vi "9082 NIVS FPGA personality + 9862_9862_SEA9811_9220_IO_sim.vi"() -> ()   [LabVIEW 2012]
uses:
  <vilib>/Platform/TimedLoop/XDataNode/timing_clust.ctl
  <vilib>/Platform/TimedLoop/XDataNode/nitl_modes.ctl
  <vilib>/Platform/TimedLoop/XDataNode/wakeup.ctl
  <vilib>/rvi/Emulation/niFpgaSctlEmulationGetInTimedLoop.vi
  <vilib>/rvi/Emulation/niFpgaSctlEmulationGlobalWrite.vi
  <vilib>/rvi/interface/RandomDataEmulation/nirviRandomDataFPGAFIFO.vi
  <vilib>/rvi/interface/RandomDataEmulation/niFpgaRandomDataHandleErrors.vi
  <vilib>/rvi/Emulation/niFpgaSctlEmulationRegisterWithScheduler.vi
  <vilib>/rvi/Emulation/niFpgaSctlEmulationScheduler.vi
  <vilib>/rvi/eio/common/nirviEmuTemplateMethod_errors.vi
  <vilib>/Platform/TimedLoop/XDataNode/XDataNode.xnode
  <vilib>/rvi/DataTransferAndStorage/Container/XNode/niFpgaContainer.xnode
  <vilib>/rvi/interface/RandomDataEmulation/nirviRandomDataFpgaReadWriteTemplate.vi
  <vilib>/eio/EIONode/EIONode.xnode
  <vilib>/Platform/TimedLoop/XDataNode/XDNodeRunTimeDep.lvlib
  <vilib>/NI Veristand/FPGA/NI_VS FPGA Support.lvlib
  <userlib>/_NI VeriStand FPGA Support/NI VeriStand FPGA Clock Support/NI_VS FPGA Clock Support.lvlib
  <vilib>/eio/EIOMethodNode/EIOMethodNode.xnode
  <userlib>/FPGA Timekeeper 1.1b0/FPGA Timekeeper.lvlib
  <vilib>/eio/EIOPropertyNode/EIOPropertyNode.xnode
  <vilib>/rvi/eio/common/nirviEmuTemplatePropertyGet_errors.vi
  <vilib>/rvi/eio/common/nirviEmuTemplatePropertyGet_noerrors.vi
  <vilib>/rvi/eio/common/nirviEmuTemplatePropertySet_errors.vi
  <vilib>/rvi/eio/common/nirviEmuTemplatePropertySet_noerrors.vi
panel:
  out "element":u64
  out "9220/AI0":fxp<+/-,24,5>
  out "Counter":u32
  out "Pulse":bool
  in  "Pulse length (ms)":u32=5
  in  "AI0_threshold (V)":fxp<+/-,24,5>=5.0
  in  "FPGA Loop rate (usec)":u16=5
  out "FPGA Timekeeper time (ns)":u64
  out "FPGA Timekeeper locked":bool
  out "offset from RT time (ns)":i32
  in  "RT time (ns)":u64
  out "DMA Overflow":bool
  out "Elements in FIFO":u32
  out "Rx Status":u16 format="%016b"
  out "Rx rate us":u32
  in  "RxSimRate(mSec)":u32=5 caption="Count(mSec)"
  out "Tx Status":u8 format="%08b"
  in  "Tx Data":u32 format="%08x"
  in  "Transmit Data":bool
  in  "Rx Channel Number":u8 max=7 step=1
  in  "Rx Config Data (RCR)":u16=32 format="%04x"
  in  "Tx Config Data (TCR)":u16=8192 format="%04x"
  in  "Rx Label Filter":u8[](array[numeric])=[0, 0, 0, 0, 0, 0, 0, 0, 0, 0, 0, 0, 0, 0, 0, 0]
  in  "Configure\nchannel":bool
  in  "Finished config":bool
  in  "Generate IRQ":bool
  in  "Use External Timing":bool
  in  "Write to  RTSI":bool
  in  "Loop Rate (usec)":u32
  in  "Start":bool
  # "Configuration"
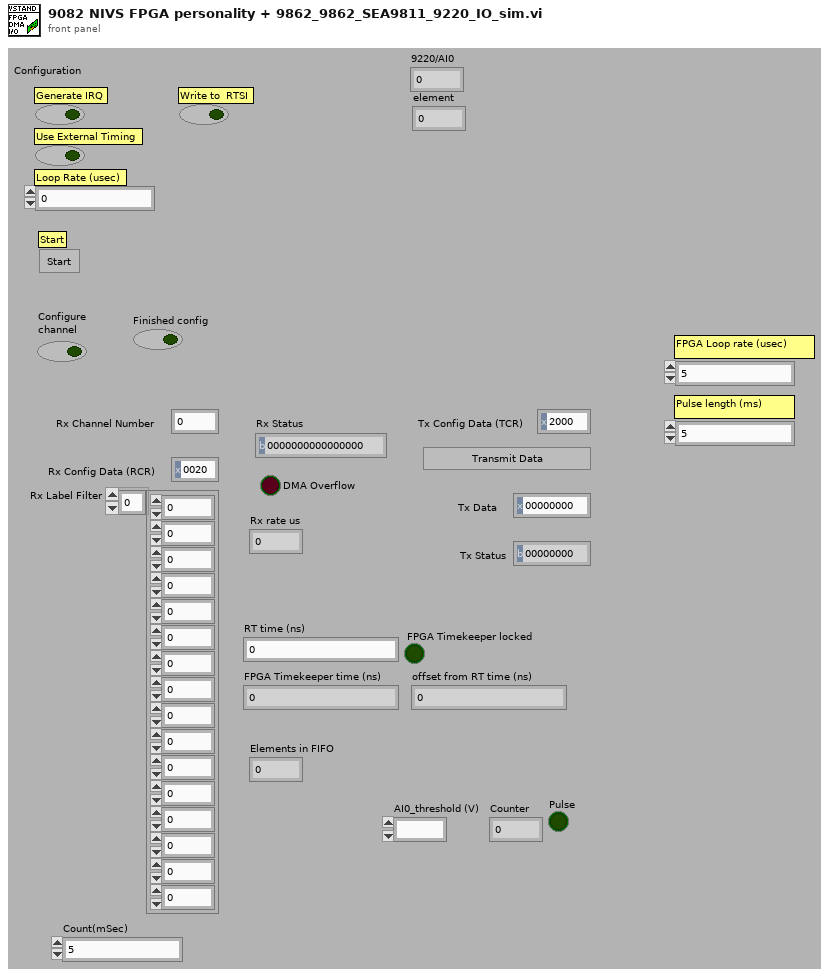
[diagram p1: front panel]
types:
  T1 = typedef "XDNodeRunTimeDep.lvlib/timing_clust.ctl" = cluster{"Expected End [f-1]":u64, "Actual End [f-1]":u64, "Finished Late? [f-1]":bool, "Expected End [i-1]":u64, "Actual End [i-1]":u64, "Finished Late? [i-1]":bool, "Expected Start [i]":u64, "Actual Start [i]":u64, "Expected Start [f]":u64, "Actual Start [f]":u64, "Source Name":string, "Structure Name":string, "Period":i64, "Deadline":i64, "Offset":i64, "Start":i64, "Priority":i32, "Timeout":i32, "Mode":T2, "Wakeup Reason":T3, "Error":errorcluster, "Source Type":string, "Secondary Source Type":string, "Global End Time":u64, "Global Start Time":u64, "Frame Duration":u64, "Iteration Duration":u64, "Assigned CPU":i32, "I/O Scan Engine Mode":u32}
  T2 = typedef "XDNodeRunTimeDep.lvlib/nitl_modes.ctl" = enum32{"No Change", "Process missed periods, maintain original phase", "Discard missed periods, maintain original phase", "Process missed periods, ignore original phase", "Discard missed periods, ignore original phase"}
  T3 = typedef "XDNodeRunTimeDep.lvlib/wakeup.ctl" = enum32{"Normal", "Aborted", "Asynchronous wakeup", "Timing source error", "Timed loop error", "Timeout"}
  T4 = cluster{"Rx Label Filter[0]":u8, "Rx Label Filter[1]":u8, "Rx Label Filter[2]":u8, "Rx Label Filter[3]":u8, "Rx Label Filter[4]":u8, "Rx Label Filter[5]":u8, "Rx Label Filter[6]":u8, "Rx Label Filter[7]":u8, "Rx Label Filter[8]":u8, "Rx Label Filter[9]":u8, "Rx Label Filter[10]":u8, "Rx Label Filter[11]":u8, "Rx Label Filter[12]":u8, "Rx Label Filter[13]":u8, "Rx Label Filter[14]":u8, "Rx Label Filter[15]":u8}
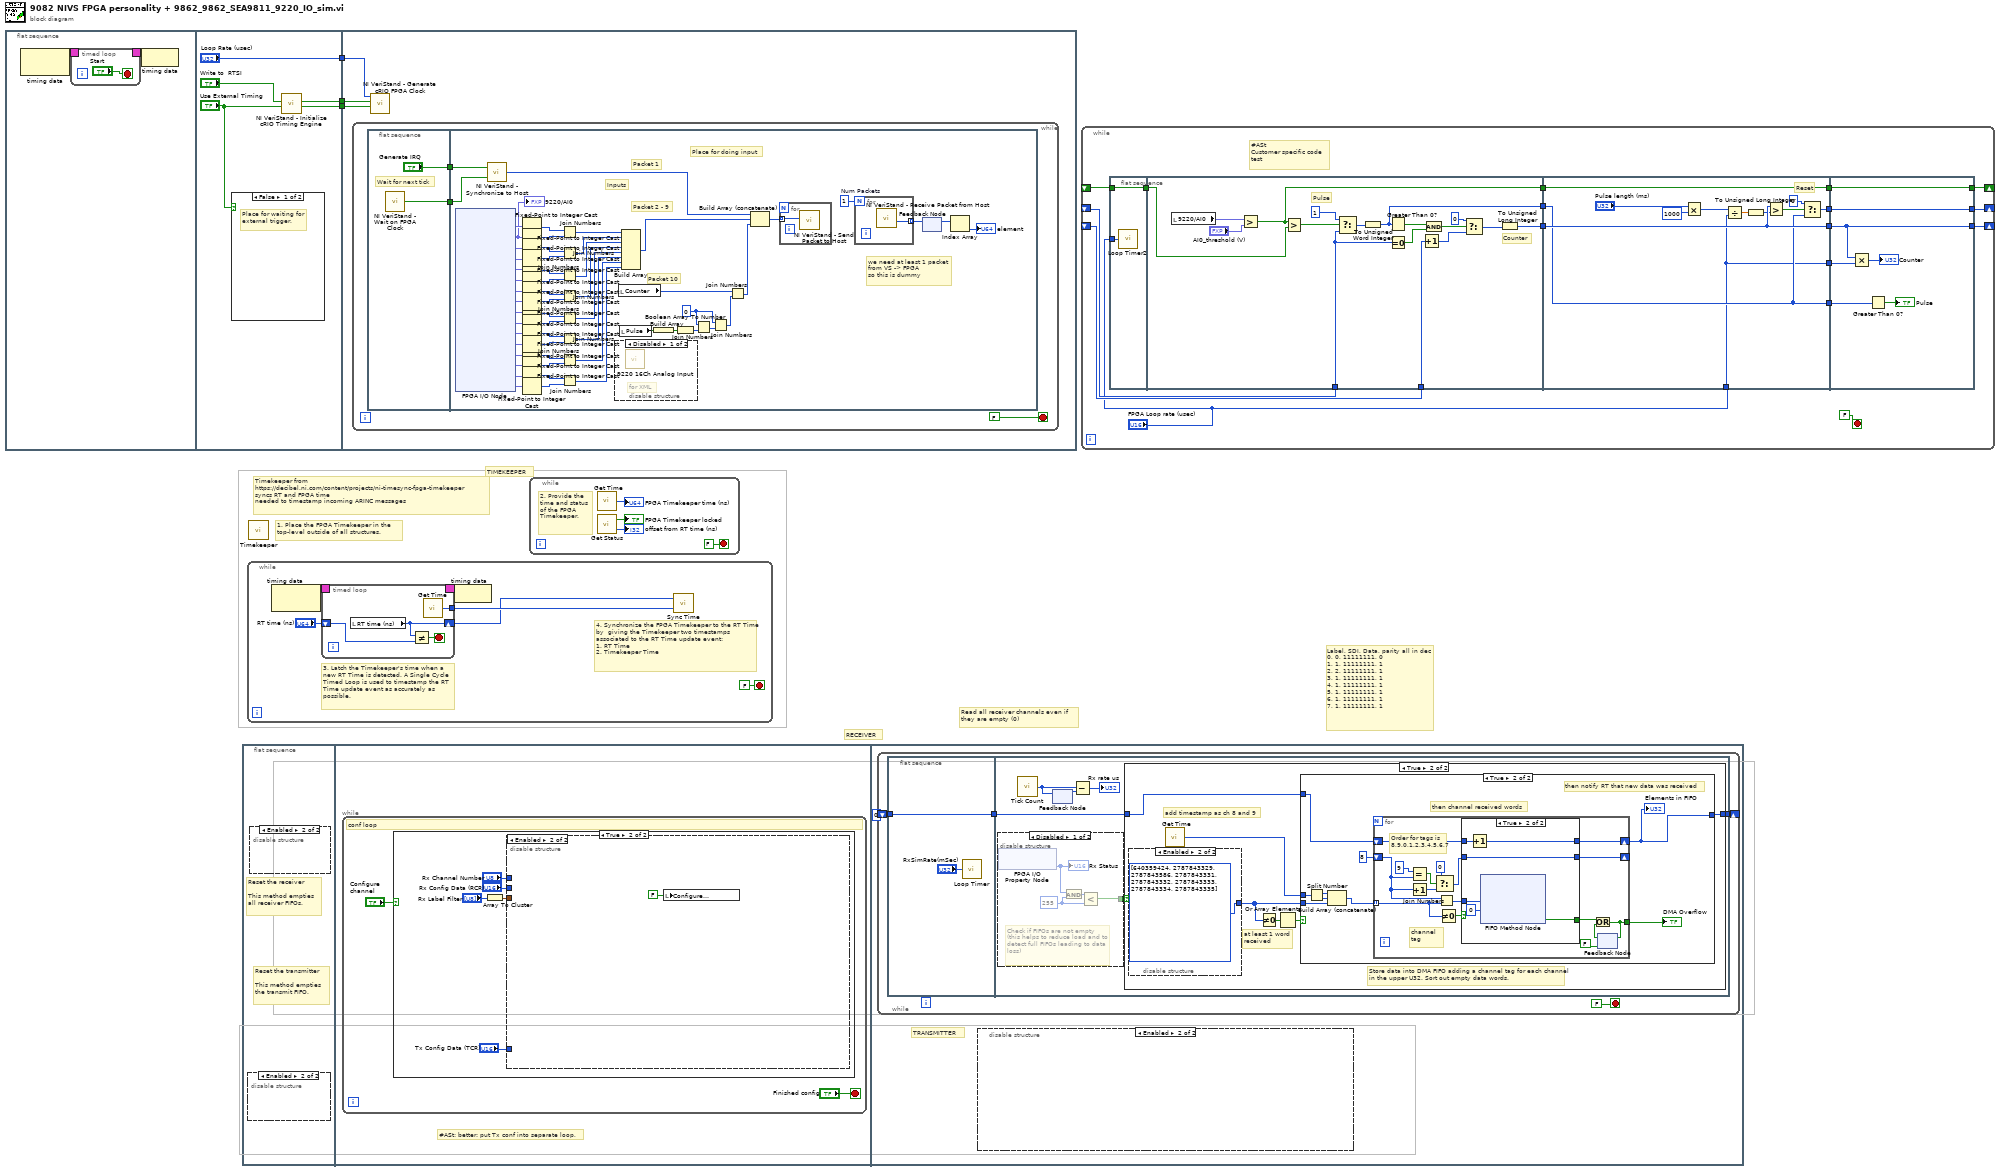
[diagram p0: block diagram]
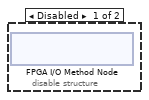
[diagram p2: hidden frame]
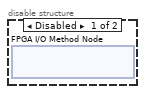
[diagram p3: hidden frame]
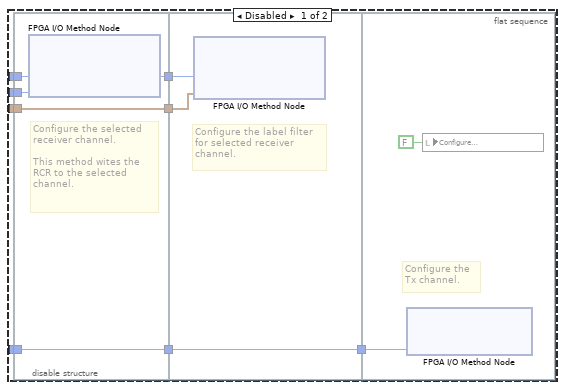
[diagram p5: hidden frame]
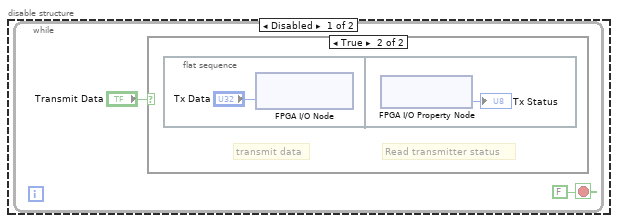
[diagram p6: hidden frame]
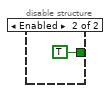
[diagram p8: hidden frame]
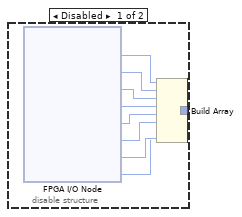
[diagram p10: hidden frame]
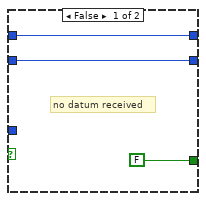
[diagram p12: hidden frame]
diagram:
  # "Label, SDI, Data, parity all in dec\n0, 0, 11111111, 0 \n1, 1, 11111111, 1 \n2, 2, 11111111, 1\n3, 1, 11111111, 1 \n4, 1, 11111111, 1 \n5, 1, 11111111, 1 \n6, 1, 11111111, 1 \n7, 1, 11111111, 1"
  # "Read all receiver channels even if they are empty (0)"
  # "TIMEKEEPER"
  # "Timekeeper from\nhttps://decibel.ni.com/content/projects/ni-timesync-fpga-timekeeper\nsyncs RT and FPGA time\nneeded to timestamp incoming ARINC messages"
  # "1. Place the FPGA Timekeeper in the top-level outside of all structures."
  # "RECEIVER"
  n1 = flat-sequence {
    tunnel: [w12] -> w3
    tunnel: ["Loop Rate (usec)"] -> w2
    tunnel: [w11] -> w1
    tunnel: w3 -> [w18]
    tunnel: w2 -> [w17]
    tunnel: w1 -> [w16]
    frame #0 {
      n2 = node-c288() -> (w5:T1)  [unwired: 1 out]
      n3 = timed-loop {
        timing: w5 -> [_]
        timing-out: [_] -> w4
        stop <- "Start" stop-if-true
      }
      n4 = node-c288(w4) -> ()
    }
    frame #1 {
      n5 = case shown="False" "Use External Timing" {
        frame False {
          # "Place for waiting for external trigger."
        }
        frame True {
          # "Do not wait on trigger when externally timed."
        }
      }
      n6 = call <userlib>:"NI VeriStand - Initialize cRIO Timing Engine.vi"("Use External Timing In"="Use External Timing", "Write to  RTSI In"="Write to  RTSI") -> ("Use External Timing Out"=w12:bool, "Write to  RTSI Out"=w11:bool)  [unwired: 8 in]
    }
    frame #2 {
      n7 = while {
        stop <- FALSE stop-if-true
        n8 = flat-sequence {
          tunnel: ["Generate IRQ"] -> w20
          tunnel: [w22] -> w19
          tunnel: w20 -> [w80]
          tunnel: w19 -> [w79]
          frame #0 {
            # "Wait for next tick"
            n9 = call <userlib>:"NI VeriStand - Wait on FPGA Clock.vi"() -> ("Clock Ticked"=w22:bool)
          }
          frame #1 {
            w27 = 1  # Num Packets
            w30 = u8 0 ("hi")
            # "we need at least 1 packet\nfrom VS -> FPGA\nso this is dummy"
            # "Packet 10"
            # "Packet 1"
            # "Inputs"
            # "Packet 2 - 9"
            # "Place for doing input"
            n10 = xnode "FPGA I/O Node"() -> ("9220/AI1"=w38:fxp<+/-,24,5>, "9220/AI0"=w34:fxp<+/-,24,5>, "9220/AI3"=w61:fxp<+/-,24,5>, "9220/AI2"=w62:fxp<+/-,24,5>, "9220/AI5"=w63:fxp<+/-,24,5>, "9220/AI4"=w64:fxp<+/-,24,5>, "9220/AI7"=w65:fxp<+/-,24,5>, "9220/AI6"=w66:fxp<+/-,24,5>, "9220/AI9"=w67:fxp<+/-,24,5>, "9220/AI8"=w68:fxp<+/-,24,5>, "9220/AI11"=w69:fxp<+/-,24,5>, "9220/AI10"=w70:fxp<+/-,24,5>, "9220/AI13"=w71:fxp<+/-,24,5>, "9220/AI12"=w72:fxp<+/-,24,5>, "9220/AI15"=w73:fxp<+/-,24,5>, "9220/AI14"=w74:fxp<+/-,24,5>)  [unwired: 16 in, 16 out]
            "9220/AI0" <- w34
            n11 = call <userlib>:"NI VeriStand - Synchronize to Host.vi"("Clock Ticked"=w79, "Generate IRQ"=w80) -> ("Is Late?"=w78:u64)
            n12 = Fixed-Point to Integer Cast(1:w38) -> (0:w39:i32)
            n13 = Fixed-Point to Integer Cast(1:w34) -> (0:w40:i32)
            n14 = Fixed-Point to Integer Cast(1:w61) -> (0:w41:i32)
            n15 = Fixed-Point to Integer Cast(1:w62) -> (0:w42:i32)
            n16 = Fixed-Point to Integer Cast(1:w63) -> (0:w46:i32)
            n17 = Fixed-Point to Integer Cast(1:w64) -> (0:w45:i32)
            n18 = Fixed-Point to Integer Cast(1:w65) -> (0:w44:i32)
            n19 = Fixed-Point to Integer Cast(1:w66) -> (0:w43:i32)
            n20 = Fixed-Point to Integer Cast(1:w67) -> (0:w47:i32)
            n21 = Fixed-Point to Integer Cast(1:w68) -> (0:w48:i32)
            n22 = Fixed-Point to Integer Cast(1:w69) -> (0:w49:i32)
            n23 = Fixed-Point to Integer Cast(1:w70) -> (0:w50:i32)
            n24 = Fixed-Point to Integer Cast(1:w71) -> (0:w54:i32)
            n25 = Fixed-Point to Integer Cast(1:w72) -> (0:w53:i32)
            n26 = Fixed-Point to Integer Cast(1:w73) -> (0:w52:i32)
            n27 = Fixed-Point to Integer Cast(1:w74) -> (0:w51:i32)
            n28 = Join Numbers(hi=w39, lo=w40) -> ((hi.lo)=w37:u64)
            n29 = Join Numbers(hi=w46, lo=w45) -> ((hi.lo)=w55:u64)
            n30 = Join Numbers(hi=w47, lo=w48) -> ((hi.lo)=w57:u64)
            n31 = Join Numbers(hi=w54, lo=w53) -> ((hi.lo)=w59:u64)
            n32 = Join Numbers(hi=w41, lo=w42) -> ((hi.lo)=w36:u64)
            n33 = Join Numbers(hi=w44, lo=w43) -> ((hi.lo)=w56:u64)
            n34 = Join Numbers(hi=w49, lo=w50) -> ((hi.lo)=w58:u64)
            n35 = Join Numbers(hi=w52, lo=w51) -> ((hi.lo)=w60:u64)
            n36 = disable-structure shown="Disabled" {
              frame Disabled {
                # "for XML"
                n37 = call <userlib>:"9220 16Ch Analog Input.vi"() -> ()  [unwired: 1 in, 1 out]
              }
              frame Enabled {
              }
            }
            n38 = local read "Counter"() -> (w76:u32)
            n39 = local read "Pulse"() -> (w29:bool)
            n40 = Build Array(w37, w36, w55, w56, w57, w58, w59, w60) -> (w35:u64[])
            n41 = Build Array(w29) -> (w33:bool[])
            n42 = Boolean Array To Number(Boolean array=w33) -> (number=w32:u8)
            n43 = Join Numbers(hi=w30, lo=w32) -> ((hi.lo)=w31:u16)
            n44 = Join Numbers(hi=w30, lo=w31) -> ((hi.lo)=w28:u32)
            n45 = Join Numbers(hi=w76, lo=w28) -> ((hi.lo)=w75:u64)
            n46 = Build Array (concatenate)(w78, w35, w75) -> (w77:u64[])
            n47 = for {
              tunnel: w77 -> [w82] mode=indexing
              n48 = call <vilib>:"NI VeriStand - Send Packet to Host.vi"("Element"=w82) -> ()  [unwired: 2 in, 9 out]
            }
            n49 = for {
              N: w27 -> [_]
              tunnel: [w81] -> w25 mode=indexing
              n50 = call <vilib>:"NI VeriStand - Receive Packet from Host.vi"() -> ("Element"=w81:u64)  [unwired: 2 in, 9 out]
            }
            n51 = feedback #1() -> (w26:u64[])  [unwired: 1 in]
            n52 = feedback-in #1(w25) -> ()
            n53 = Index Array(array=w26) -> (element=→"element":u64)  [unwired: 1 in]
          }
        }
      }
      n54 = call <userlib>:"NI VeriStand - Generate cRIO FPGA Clock.vi"("Use External Timing"=w18, "Write to  RTSI"=w16, "Loop Rate (usec)"=w17) -> ()  [unwired: 9 in]
    }
  }
  n55 = flat-sequence {
    frame #0 {
      # "Reset the transmitter\n\nThis method empties\nthe transmit FIFO."
      # "Reset the receiver\n\nThis method empties\nall receiver FIFOs."
      n56 = disable-structure shown="Enabled" {
        frame Disabled {
          n57 = xnode "FPGA I/O Method Node"() -> ()  [unwired: 1 in, 1 out]
        }
        frame Enabled {
        }
      }
      n58 = disable-structure shown="Enabled" {
        frame Disabled {
          n59 = xnode "FPGA I/O Method Node"() -> ()  [unwired: 1 in, 1 out]
        }
        frame Enabled {
        }
      }
    }
    frame #1 {
      # "#ASt: better: put Tx conf into separate loop,"
      n60 = while {
        stop <- "Finished config" stop-if-true
        # "conf loop"
        n61 = case shown="True" "Configure\nchannel" {
          frame False {
          }
          frame True {
            n62 = Array To Cluster(array="Rx Label Filter") -> (cluster=w85:T4)
            n63 = disable-structure shown="Enabled" {
              disable-tunnel: "Rx Channel Number" -> [w93 _]
              disable-tunnel: "Rx Config Data (RCR)" -> [w92 _]
              disable-tunnel: w85 -> [w91 _]
              disable-tunnel: "Tx Config Data (TCR)" -> [w90 _]
              frame Disabled {
                n64 = flat-sequence {
                  tunnel: w93 -> [w101]
                  tunnel: [w101] -> w97
                  tunnel: w92 -> [w100]
                  tunnel: [w99] -> w96
                  tunnel: w91 -> [w99]
                  tunnel: w90 -> [w98]
                  tunnel: [w98] -> w95
                  tunnel: w97 -> [w104]
                  tunnel: w96 -> [w103]
                  tunnel: [w102] -> w94
                  tunnel: w95 -> [w102]
                  tunnel: w94 -> [w106]
                  frame #0 {
                    # "Configure the selected\nreceiver channel.\n\nThis method wites the\nRCR to the selected\nchannel."
                    n65 = xnode "FPGA I/O Method Node"("Channel Number"=w101, "Control Register"=w100) -> ()  [unwired: 1 in, 1 out]
                  }
                  frame #1 {
                    # "Configure the label filter\nfor selected receiver\nchannel."
                    n66 = xnode "FPGA I/O Method Node"("Channel Number"=w104, "Label Filter"=w103) -> ()  [unwired: 1 in, 1 out]
                  }
                  frame #2 {
                    # "Configure the\nTx channel."
                    n67 = xnode "FPGA I/O Method Node"("Control Register"=w106) -> ()  [unwired: 1 in, 1 out]
                    n68 = local write "Configure\nchannel"(FALSE ("Configure\nchannel")) -> ()
                  }
                }
              }
              frame Enabled {
                n69 = local write "Configure\nchannel"(FALSE ("Configure\nchannel")) -> ()
              }
            }
          }
        }
      }
    }
    frame #2 {
      # "TRANSMITTER"
      n70 = while {
        shift-right: [w114] -> _
        shift-left: u32 0 -> [w115]
        stop <- FALSE stop-if-true
        n71 = flat-sequence {
          tunnel: w115 -> [w118]
          tunnel: [w118] -> w113
          tunnel: [w122] -> w114
          tunnel: w113 -> [w123]
          frame #0 {
            n72 = call "Loop Timer"("Count(mSec)"="RxSimRate(mSec)") -> ()  [unwired: 1 out]
          }
          frame #1 {
            n73 = disable-structure shown="Disabled" {
              disable-tunnel: [w125 TRUE] -> w124
              frame Disabled {
                w126 = u16 255 ("y")
                # "Check if FIFOs are not empty\n(this helps to reduce load and to detect full FIFOs leading to data loss)"
                n74 = xnode "FPGA I/O Property Node"() -> ("Rx Status"=w128:u16)  [unwired: 1 in, 1 out]
                "Rx Status" <- w128
                n75 = And(x=w128, y=w126) -> (x .and. y?=w127:u16)
                n76 = Less?(x=w127, y=w126) -> (x < y?=w125:bool)
              }
              frame Enabled {
              }
            }
            n77 = call "Tick Count"() -> ("Tick Count(uSec)"=w119:u32)
            n78 = feedback #2() -> (w120:u32)  [unwired: 1 in]
            n79 = feedback-in #2(w119) -> ()
            n80 = Subtract(x=w119, y=w120) -> (x-y=→"Rx rate us":u32)
            n81 = case shown="True" w124 {
              tunnel: w123 -> [w130 w136]
              tunnel: [w130 w135] -> w122
              frame False {
              }
              frame True {
                # "add timestamp as ch 8 and 9"
                # "at least 1 word\nreceived"
                # "Store data into DMA FIFO adding a channel tag for each channel in the upper U32. Sort out empty data words."
                n82 = disable-structure shown="Enabled" {
                  disable-tunnel: [w137 u32[] [640359424, 2787843329, 2787843586, 2787843331, 2787843332, 2787843333, 2787843334, 2787843335]] -> w134
                  frame Disabled {
                    n83 = xnode "FPGA I/O Node"() -> ("Mod1/Rx0"=w139:u32, "Mod1/Rx1"=w140:u32, "Mod1/Rx2"=w141:u32, "Mod1/Rx3"=w142:u32, "Mod1/Rx4"=w143:u32, "Mod1/Rx5"=w144:u32, "Mod1/Rx6"=w145:u32, "Mod1/Rx7"=w138:u32)  [unwired: 8 in, 8 out]
                    n84 = Build Array(w139, w140, w141, w142, w143, w144, w145, w138) -> (w137:u32[])
                  }
                  frame Enabled {
                  }
                }
                n85 = call <userlib>:"Get Time.vi"() -> ("time (ns)"=w131:u64)
                n86 = Not Equal To 0?(x=w134) -> (x != 0?=w133:bool[])
                n87 = Or Array Elements(Boolean array=w133) -> (logical OR=w132:bool)
                n88 = case shown="True" w132 {
                  tunnel: w136 -> [w147 w148]
                  tunnel: [w147 w156] -> w135
                  tunnel: w134 -> [_ w153]
                  tunnel: w131 -> [_ w149]
                  frame False {
                  }
                  frame True {
                    # "then notify RT that new data was received"
                    # "then channel received words"
                    n89 = Split Number(x=w149) -> (hi(x)=w151:u32, lo(x)=w150:u32)
                    n90 = Build Array (concatenate)(w151, w150, w153) -> (w152:u32[])
                    n91 = for {
                      tunnel: w152 -> [w164] mode=indexing
                      tunnel: [w169] -> w155
                      shift-right: [w165] -> w156
                      shift-left: w148 -> [w166]
                      shift-right: [w157] -> _
                      shift-left: u32 8 ("hi") -> [w161]
                      # "Order for tags is\n8,9,0,1,2,3,4,5,6,7"
                      # "channel\ntag"
                      n92 = Equal?(x=u32 9, y=w161) -> (x = y?=w162:bool)
                      n93 = Increment(x=w161) -> (x+1=w163:u32)
                      n94 = Select(t=u32 0, s=w162, f=w163) -> (s? t:f=w158:u32)
                      n95 = Join Numbers(hi=w161, lo=w164) -> ((hi.lo)=w167:u64)
                      n96 = Not Equal To 0?(x=w164) -> (x != 0?=w168:bool)
                      n97 = case shown="True" w168 {
                        tunnel: [FALSE ("Timed Out?") w181] -> w170
                        tunnel: w167 -> [_ w178]
                        tunnel: w166 -> [w174 w180]
                        tunnel: [w174 w179] -> w165
                        tunnel: w158 -> [w173 w176]
                        tunnel: [w173 w176] -> w157
                        frame False {
                          # "no datum received"
                        }
                        frame True {
                          n98 = Increment(x=w180) -> (x+1=w179:u32)
                          n99 = xnode ("FIFO Method Node")("Element"=w178, "Timeout"=0) -> ("Timed Out?"=w181:bool)  [unwired: 1 in, 1 out]
                        }
                      }
                      n100 = feedback #3(FALSE) -> (w171:bool)
                      n101 = Or(x=w170, y=w171) -> (x .or. y?=w169:bool)
                      n102 = feedback-in #3(w169) -> ()
                    }
                    "DMA Overflow" <- w155
                    "Elements in FIFO" <- w156
                  }
                }
              }
            }
          }
        }
      }
      n103 = disable-structure shown="Enabled" {
        frame Disabled {
          n104 = while {
            stop <- FALSE stop-if-true
            n105 = case shown="True" "Transmit Data" {
              frame False {
              }
              frame True {
                # "Read transmitter status"
                # "transmit data"
                n106 = flat-sequence {
                  frame #0 {
                    n107 = xnode "FPGA I/O Node"("Mod1/Tx0"="Tx Data") -> ()  [unwired: 1 in, 1 out]
                  }
                  frame #1 {
                    n108 = xnode "FPGA I/O Property Node"() -> ("Tx Status"=→"Tx Status":u8)  [unwired: 1 in, 1 out]
                  }
                }
              }
            }
          }
        }
        frame Enabled {
        }
      }
    }
  }
  n109 = while {
    stop <- FALSE stop-if-true
    # "3. Latch the Timekeeper's time when a new RT Time is detected. A Single Cycle Timed Loop is used to timestamp the RT Time update event as accurately as possible."
    # "4. Synchronize the FPGA Timekeeper to the RT Time by  giving the Timekeeper two timestamps associated to the RT Time update event:\n1. RT Time\n2. Timekeeper Time"
    n110 = node-c288() -> (w187:T1)  [unwired: 1 in]
    n111 = timed-loop {
      timing: w187 -> [_]
      timing-out: [_] -> w186
      shift-right: [w188] -> w182
      shift-left: "RT time (ns)" -> [w189]
      tunnel: [w191] -> w185
      stop <- w190 stop-if-true
      n112 = local read "RT time (ns)"() -> (w188:u64)
      n113 = Not Equal?(x=w188, y=w189) -> (x != y?=w190:bool)
      n114 = call <userlib>:"Get Time.vi"() -> ("time (ns)"=w191:u64)
    }
    n115 = node-c288(w186) -> ()
    n116 = call <userlib>:"Sync Time.vi"("FPGA Timekeeper time (ns)"=w185, "time reference time (ns)"=w182) -> ()
  }
  n117 = call <userlib>:"Timekeeper.vi"() -> ()  [unwired: 12 in]
  n118 = while {
    stop <- FALSE stop-if-true
    # "2. Provide the time and status of the FPGA Timekeeper."
    n119 = call <userlib>:"Get Time.vi"() -> ("time (ns)"=→"FPGA Timekeeper time (ns)":u64)
    n120 = call <userlib>:"Get Status.vi"() -> ("FPGA Timekeeper locked"=→"FPGA Timekeeper locked":bool, "offset from time reference"=→"offset from RT time (ns)":i32)
  }
  n121 = while {
    shift-right: [w215] -> _
    shift-left: _ -> [w214]
    shift-right: [w213] -> _
    shift-left: _ -> [w208]
    shift-right: [w209] -> _
    shift-left: _ -> [w207]
    stop <- FALSE stop-if-true
    # "#ASt\nCustomer specific code\ntest"
    n122 = flat-sequence {
      tunnel: w214 -> [w218]
      tunnel: [w218] -> w206
      tunnel: "FPGA Loop rate (usec)" -> [w217]
      tunnel: [w220] -> w212
      tunnel: [w223] -> w211
      tunnel: [w222] -> w210
      tunnel: w208 -> [w226]
      tunnel: w207 -> [w225]
      tunnel: w206 -> [w235]
      tunnel: w210 -> [w243]
      tunnel: w211 -> [w237]
      tunnel: w212 -> [w247]
      tunnel: "FPGA Loop rate (usec)" -> [w236]
      tunnel: [w247] -> w204
      tunnel: [w246] -> w203
      tunnel: [w243] -> w202
      tunnel: [w237] -> w201
      tunnel: [w236] -> w200
      tunnel: [w251] -> w209
      tunnel: [w253] -> w213
      tunnel: [w254] -> w215
      tunnel: w204 -> [w254]
      tunnel: w203 -> [w253]
      tunnel: w202 -> [w251]
      tunnel: w201 -> [w252]
      tunnel: w200 -> [w250]
      frame #0 {
        n123 = call "Loop Timer2"("Count(uSec)"=w217) -> ()  [unwired: 1 out]
      }
      frame #1 {
        # "Pulse"
        # "Counter"
        n124 = local read "9220/AI0"() -> (w219:fxp<+/-,24,5>)
        n125 = Greater?(x=w219, y="AI0_threshold (V)") -> (0:w220:bool)
        n126 = Greater?(x=w220, y=w235) -> (0:w234:bool)
        n127 = Select(t=u8 1, s=w234, f=w226) -> (s? t:f=w232:u16)
        n128 = To Unsigned Word Integer(number=w232) -> (unsigned 16bit integer=w223:u16)
        n129 = Greater Than 0?(x=w223) -> (x > 0?=w231:bool)
        n130 = Equal To 0?(x=w226) -> (x = 0?=w230:bool)
        n131 = Increment(x=w225) -> (x+1=w227:u32)
        n132 = And(x=w231, y=w230) -> (x .and. y?=w229:bool)
        n133 = Select(t=u8 0, s=w229, f=w227) -> (s? t:f=w224:u32)
        n134 = To Unsigned Long Integer(number=w224) -> (unsigned 32bit integer=w222:u32)
      }
      frame #2 {
        # "Reset"
        n135 = Multiply(x="Pulse length (ms)", y=i16 1000) -> (x*y=w240:u32)
        n136 = Divide(x=w240, y=w236) -> (x/y=w238:sgl)
        n137 = To Unsigned Long Integer(number=w238) -> (unsigned 32bit integer=w239:u32)
        n138 = Greater?(x=w243, y=w239) -> (0:w244:bool)
        n139 = Select(t=u8 0, s=w244, f=w237) -> (s? t:f=w246:u16)
      }
      frame #3 {
        n140 = Multiply(x=w251, y=w250) -> (x*y=→"Counter":u32)
        n141 = Greater Than 0?(x=w252) -> (x > 0?=→"Pulse":bool)
      }
    }
  }
